vi "main_control_combo_reframe.vi"() -> ()   [LabVIEW 2019]
doc: "The Basic Serial Read and Write example performs a Serial Port Read, a Serial Port Write, or a combination of these actions. The user selects the actions (read or write) on the front panel. If both are selected, the VI will write the data first, read data, and then close the VISA session that is opened to the port. This VI will wait until the specified number of bytes is received at the port. Only the number of bytes specified will be read.\n\nINSTRUCTIONS:\n1) Select the serial resource and configuration parameters (baud rate, data bits, parity, stop bits, flow control).\n2) Select the operations to be performed. \n3) Connect the serial port to your device. If no device is available, perform a loopback test by doing one of the following. Short pins 2 and 3 on a RS-232 cable or short pin 4 to pin 8 and pin 5 to pin 9 on a RS-485/422 cable. \n4) Run the VI to see the data read. (The \"read string\" will match the \"string to write\" if a loopback test was performed.)\n\nNote: The parameters set for the serial port must match the parameters of the connected instrument or device. In this example, the bytes to read parameter specifies the number of bytes that the serial port reads. If there were more bytes at the port than the number specified in bytes to read, those bytes would not be read. Also, if you specify to read more bytes than the number of bytes actually read, you might receive a timeout error message.\n\nOn the block diagram, the Configure Serial Port VI sets the configuration parameters. The front panel displays the controls used to configure the basic parameters, such as baud rate, data bits, and parity. Constants configure the other parameters the user probably does not need set. After the VISA Configure Serial Port VI opens the VISA session and configures the port, the VI passes the VISA resource name to other VIs that perform operations on that VISA resource. The VISA Write function sends a command to the serial device and the VISA Read function returns data based on the command. The VISA Close function then closes the reference to the serial device. It is important to close the reference; otherwise communication through with that port through protocols other than VISA might not be possible."
uses:
  <vilib>/Instr/_visa.llb/VISA Configure Serial Port (Instr).vi
  <vilib>/Utility/file.llb/Read Delimited Spreadsheet (string).vi
  Keithley/Keithley 24XX/Public/Data/Read (Single Point).vi
  Keithley/Keithley 24XX/Keithley 24XX.lvlib
  <resource>/objmgr/ni.var.rc
panel:
  in  "Times to Run":i32
  out "DeltaPS output voltage":string
  out "SEH LV PS actual voltage":string
  out "Inverter PS actual voltage":string
  out "chiller actual temperature":string
  out "COMBO COMMAND":string
  in  "stop reading script":bool
  out "concatenated string":string
  out "dewpoint":string
  out "temperature":string
  out "humidity":string
  out "n2 flow temperature":string
  out "dewpoint":string
  out "From Linux Box":string
  in  "Voltage Manual Range (1.0) 2":dbl=1.0
  in  "Current Manual Range (1.0) 2":dbl=1.0
  in  "Resistance Manual Range (1.0) 2":dbl=1.0
  in  "Enable Voltage Auto Range (T:Enable) 2":bool=TRUE
  in  "Enable Current Auto Range (T:Enable) 2":bool=TRUE
  in  "Enable Resistance Auto Range (T:Enable) 2":bool=TRUE
  out "Voltage 3":sgl
  out "Current 3":sgl
  out "Resistance 2":sgl
  out "Current Micro 2":sgl
  out "Command Log and Output":string
  out "all rows":string[][](array[string])
  out "current command":string[](array[string])
  in  "file path (dialog if empty) 2":path
  in  "Read Script":bool
  out "relay TTi":errorcluster
  out "LV TTi":errorcluster
  out "Chiller":errorcluster
  out "N2 temperature > dew point + 2C":bool
  in  "File Path of rotonic datalog":path
  out "time humidity temporature dewpoint":string[](array[string])
  in  "Quit":bool
  # "Keithley Powersupply"
  # "µA"
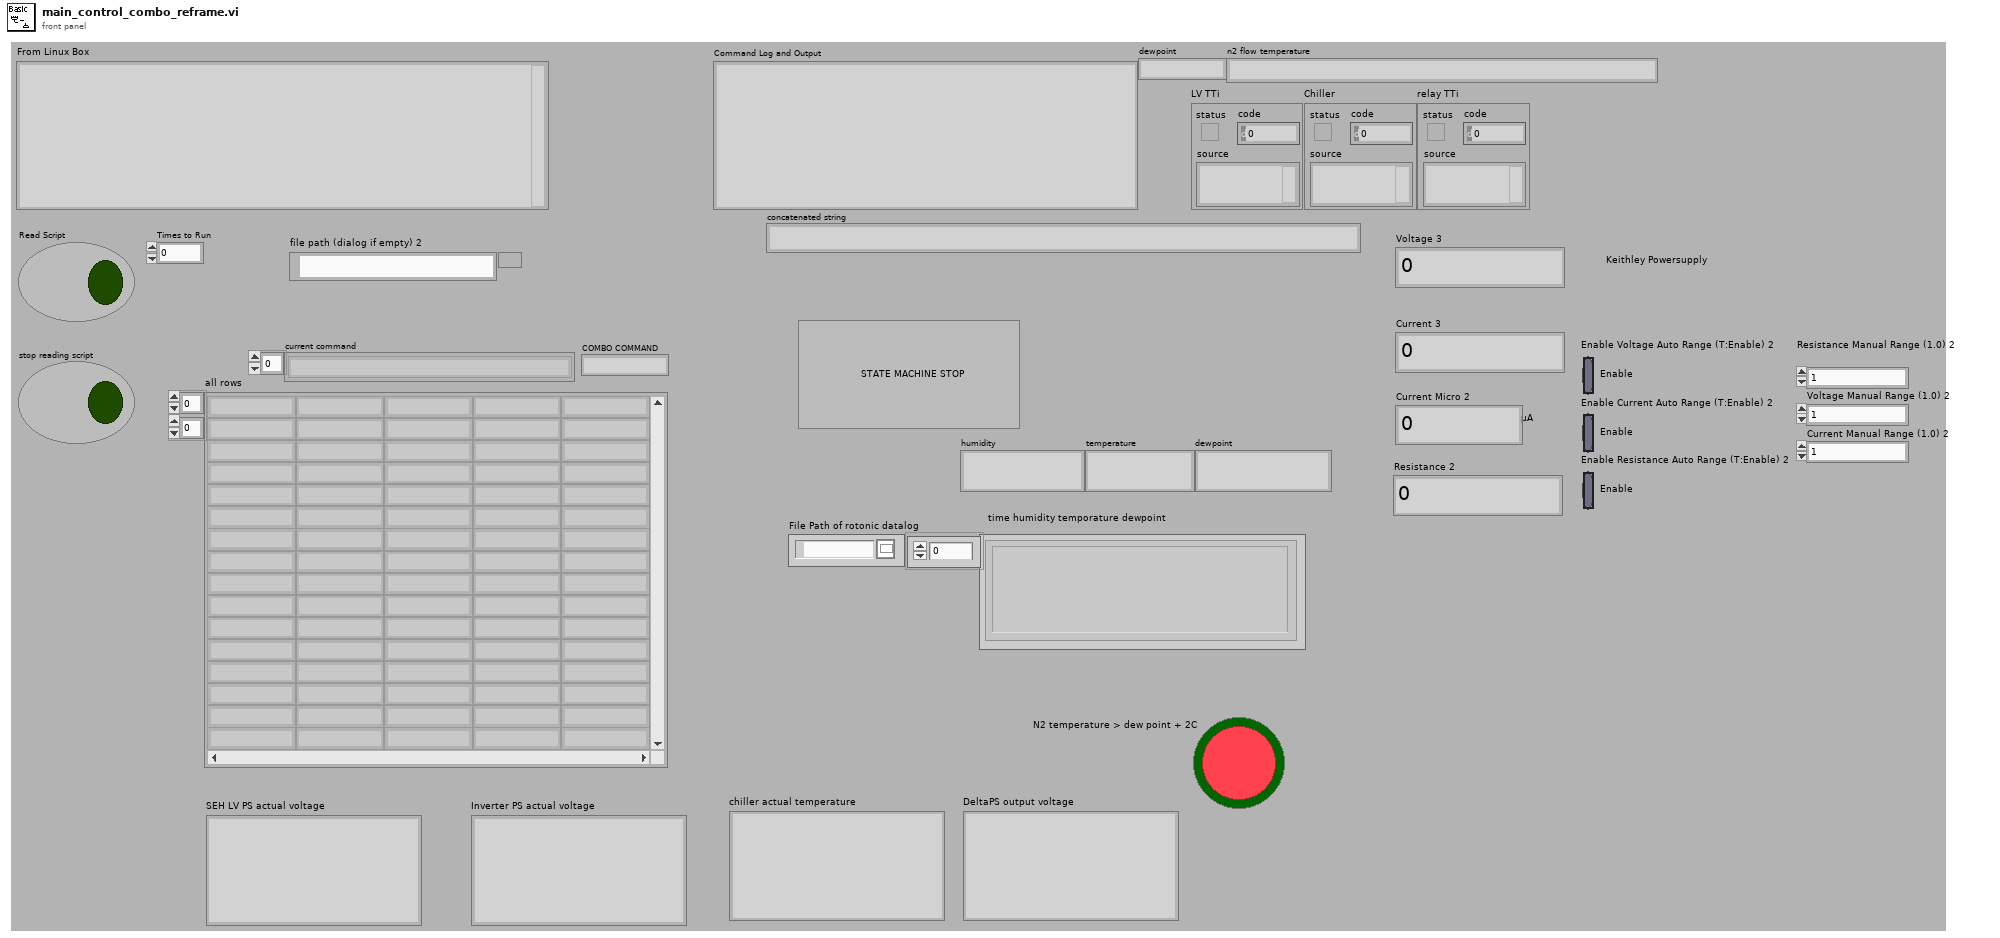
[diagram p1: front panel]
types:
  T1 = cluster{"Baud Rate":u32, "Parity":u16, "Data Bits":u16, "Stop Bits":u16, "Flow Control":u16}
  T2 = enum16{"open", "replace", "create", "open or create", "replace or create", "replace or create with confirmation"}
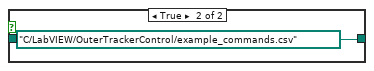
[diagram p2: hidden frame]
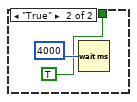
[diagram p3: hidden frame]
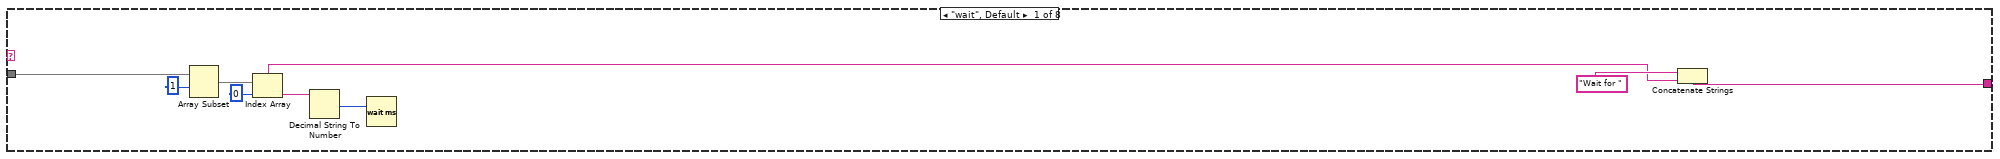
[diagram p5: hidden frame]
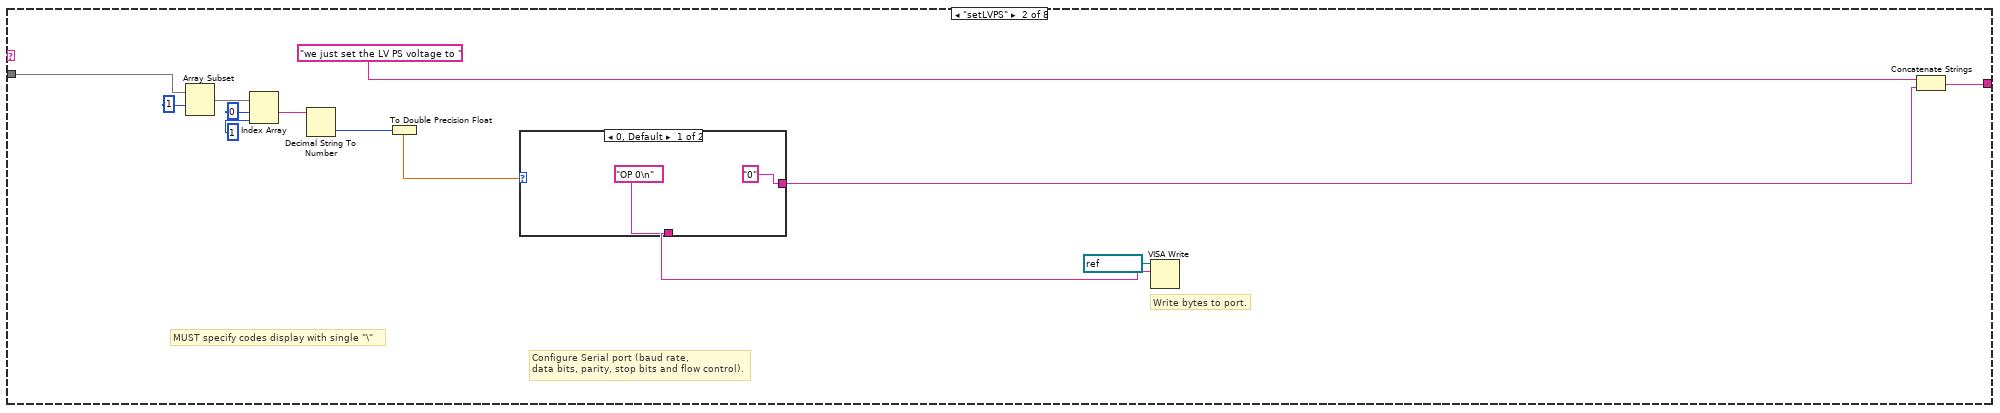
[diagram p6: hidden frame]
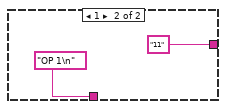
[diagram p7: hidden frame]
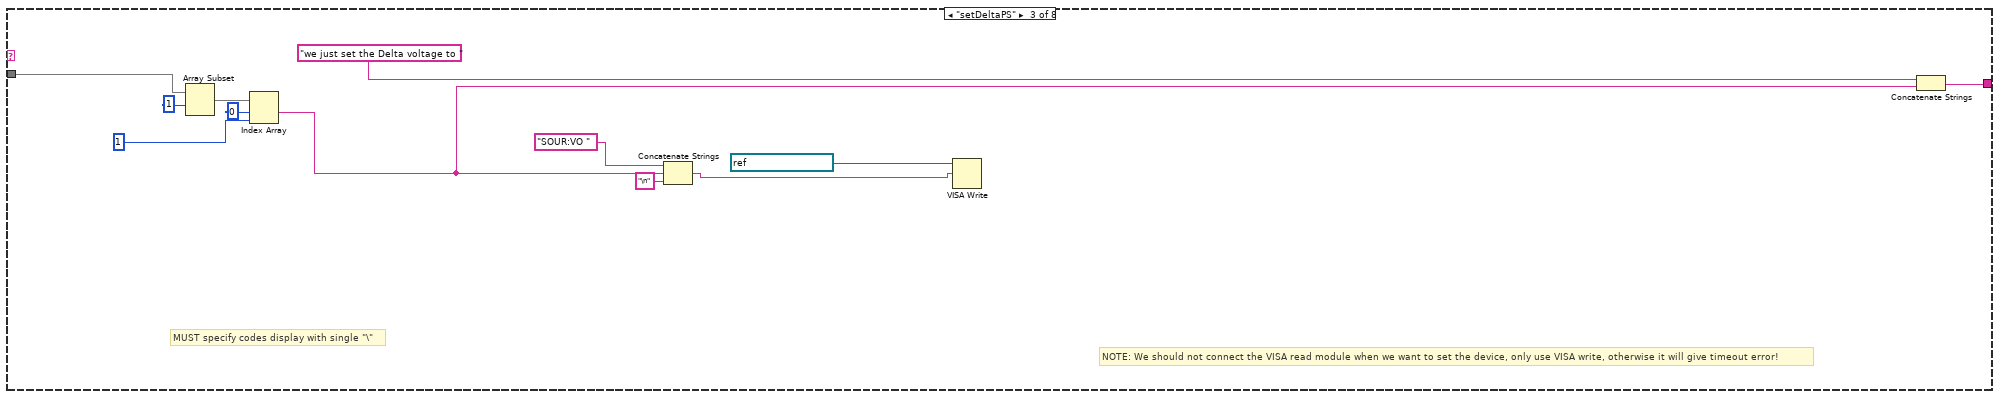
[diagram p8: hidden frame]
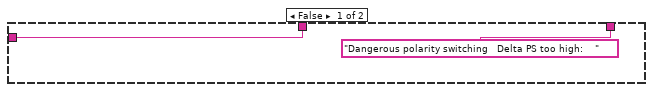
[diagram p9: hidden frame]
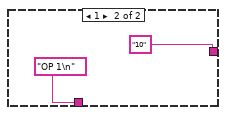
[diagram p10: hidden frame]
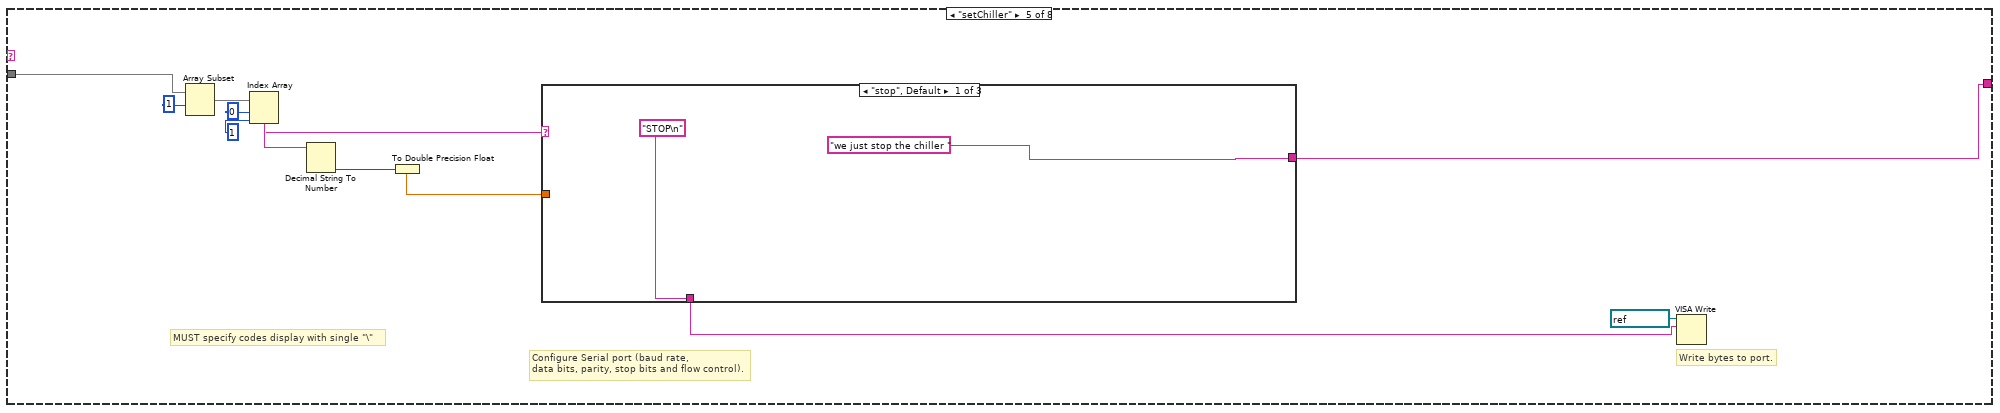
[diagram p11: hidden frame]
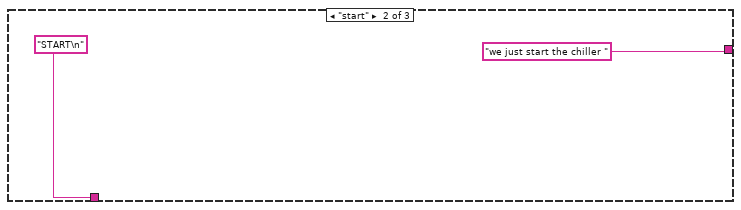
[diagram p12: hidden frame]
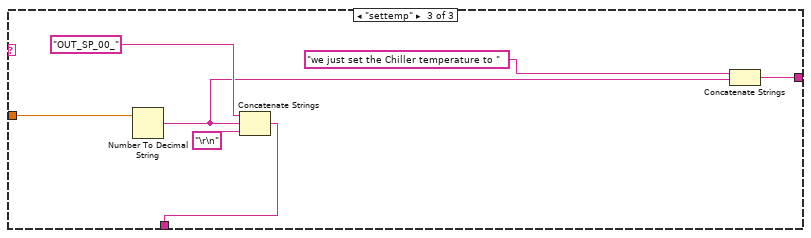
[diagram p13: hidden frame]
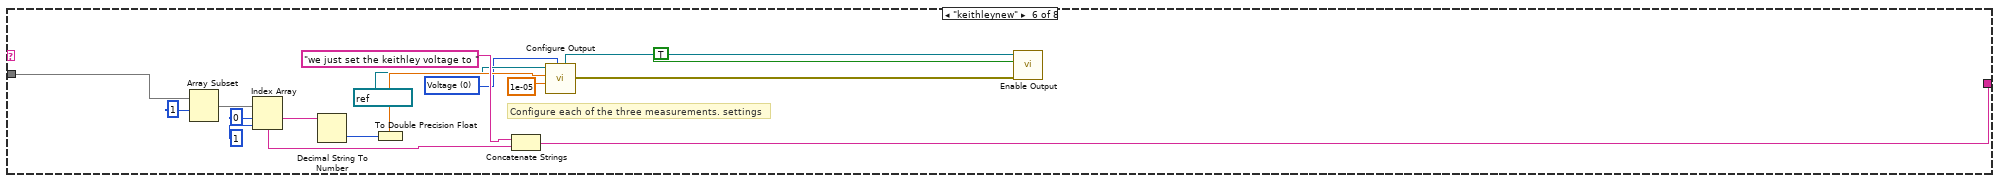
[diagram p14: hidden frame]
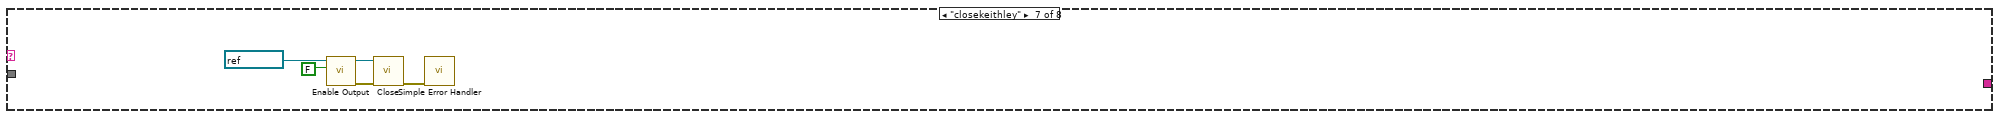
[diagram p15: hidden frame]
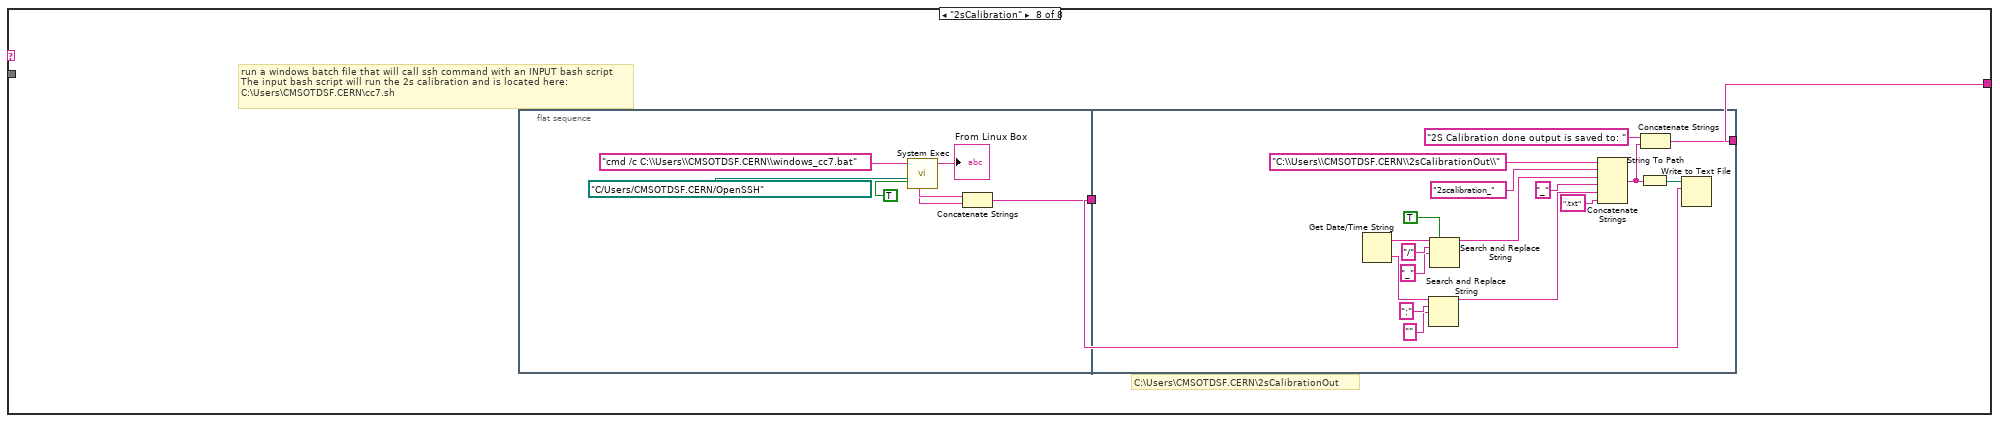
[diagram p16: hidden frame]
diagram:
  # "First save permanent values in non-volatile memory via NI - Max and the *SAV after setting it via SO:VO:MA 52 and SO:CU:MA 30    !"
  n1 = flat-sequence {
    tunnel: [w37] -> w16
    tunnel: [w36] -> w15
    tunnel: [w28] -> w14
    tunnel: [w27] -> w13
    tunnel: [w23] -> w12
    tunnel: [w22] -> w11
    tunnel: [w19] -> w10
    tunnel: [w18] -> w9
    tunnel: w16 -> [w44]
    tunnel: w15 -> [w45]
    tunnel: w14 -> [w43]
    tunnel: w13 -> [w42]
    tunnel: w12 -> [w46]
    tunnel: w11 -> [w47]
    tunnel: w10 -> [w41]
    tunnel: w9 -> [w40]
    tunnel: [w47] -> w8
    tunnel: [w46] -> w7
    tunnel: [w45] -> w6
    tunnel: [w44] -> w5
    tunnel: [w43] -> w4
    tunnel: [w42] -> w3
    tunnel: [w41] -> w2
    tunnel: [w40] -> w1
    tunnel: w8 -> [w359]
    tunnel: w7 -> [w358]
    tunnel: w6 -> [w357]
    tunnel: w5 -> [w356]
    tunnel: w4 -> [w355]
    tunnel: w3 -> [w354]
    tunnel: w2 -> [w353]
    tunnel: w1 -> [w352]
    frame #0 {
      w20 = u32 500  # timeout (10sec)
      w24 = FALSE  # Enable Termination Char (T)
      w25 = u32 3000  # timeout (10sec)
      w29 = FALSE  # Enable Termination Char (T)
      w30 = u32 3000  # timeout (10sec)
      w35 = u32 3000  # timeout (10sec)
      w33 = FALSE  # Enable Termination Char (T)
      n2 = call "Initialize.vi"("Serial Configuration"=T1 {"Baud Rate"=9600, "Parity"=0, "Data Bits"=8, "Stop Bits"=10, "Flow Control"=1}, "Reset (True)"=FALSE, "VISA resource name"=refnum<visa-resource-name> "COM1" ("VISA resource name 4")) -> ()  [unwired: 7 in, 2 out]
      n3 = call-poly "VISA Configure Serial Port"("VISA resource name"=refnum<visa-resource-name> "COM4", "timeout (10sec)"=w35, "Enable Termination\nChar (T)"=w33) -> ("VISA resource name out"=w36:refnum<visa-resource-name>, "error out"=w37:errorcluster)  [unwired: 11 in]
      n4 = VISA Open(timeout (0)=w20, VISA resource name=refnum<visa-resource-name> "GPIB0::8::INSTR") -> (VISA resource name=w19:refnum<visa-resource-name>, error out=w18:errorcluster)  [unwired: 3 in]
      n5 = call-poly "VISA Configure Serial Port"("VISA resource name"=refnum<visa-resource-name> "COM5", "timeout (10sec)"=w25, "Enable Termination\nChar (T)"=w24) -> ("VISA resource name out"=w22:refnum<visa-resource-name>, "error out"=w23:errorcluster)  [unwired: 11 in]
      n6 = call-poly "VISA Configure Serial Port"("VISA resource name"=refnum<visa-resource-name> "COM6", "timeout (10sec)"=w30, "Enable Termination\nChar (T)"=w29) -> ("VISA resource name out"=w28:refnum<visa-resource-name>, "error out"=w27:errorcluster)  [unwired: 11 in]
    }
    frame #1 {
      # "Disable Output"
      # "State machine for iterating through commands from table"
      n7 = while {
        stop <- w94 stop-if-true
        n8 = local read "Quit"() -> (w94:bool)
        n9 = case shown="True" "Read Script" {
          tunnel: "Times to Run" -> [_ w99]
          frame False {
          }
          frame True {
            n10 = Get Date/Time String() -> (date string=w122:string, time string=w120:string)  [unwired: 3 in]
            n11 = Search and Replace String(replace all?=TRUE ("replace all? (F)"), input string=w122, search string="/", replace string="_" ("replace string (\"\")")) -> (result string=w121:string)  [unwired: 4 in, 3 out]
            n12 = Search and Replace String(input string=w120, search string=":", replace string="" ("replace string (\"\")")) -> (result string=w119:string)  [unwired: 5 in, 3 out]
            n13 = Concatenate Strings("C:\\Users\\CMSOTDSF.CERN\\ExecutedCommands\\" ("string"), "command_log_" ("string"), w121, "_" ("string"), w119, ".txt" ("string")) -> (w118:string)
            n14 = String To Path(string=w118) -> (path=w108:path)
            n15 = Open/Create/Replace File(file path (use dialog)=w108, operation (0:open)=T2."replace or create") -> (refnum out=w107:refnum<file>)  [unwired: 4 in, 2 out]
            n16 = Concatenate Strings("Command Log Header for Executed CSV commands " ("text"), "\r\n") -> (w100:string)
            n17 = Set File Position(offset (in bytes) (0)=i64 0, refnum=w107, from (0:start)=enum16{"start", "end", "current"}."end") -> (refnum out=w104:refnum<file>)  [unwired: 1 in, 1 out]
            n18 = Write to Text File(file (use dialog)=w104, text=w100) -> ()  [unwired: 2 in, 3 out]
            n19 = call-poly <vilib>:"Read Delimited Spreadsheet.vi"("file path (dialog if empty)"="file path (dialog if empty) 2", "delimiter (\\t)"="," ("delimiter (\\t)")) -> ("all rows"=w97:string[][])  [unwired: 8 in, 5 out]
            n20 = flat-sequence {
              tunnel: w108 -> [w125]
              tunnel: w99 -> [w124]
              tunnel: w97 -> [w123]
              frame #0 {
                n21 = for {
                  N: w124 -> [_]
                  tunnel: w125 -> [w131]
                  tunnel: w123 -> [w130]
                  # "read table from CSV"
                  n22 = Array Size(array=w130) -> (size(s)=w128:i32[])
                  n23 = Index Array(array=w128, index #1=0 ("index"), index #2=1 ("index")) -> (element #1=w129:i32)  [unwired: 1 out]
                  n24 = for {
                    N: w129 -> [_]
                    tunnel: w130 -> [w137] mode=indexing
                    tunnel: w131 -> [w133]
                    i -> [w132]
                    stop <- w134 stop-if-true
                    n25 = flat-sequence {
                      tunnel: w137 -> [w158]
                      tunnel: w133 -> [w149]
                      tunnel: w132 -> [w146]
                      frame #0 {
                        n26 = Array Subset(array=w158) -> (w155:string[])  [unwired: 2 in]
                        "current command" <- w155
                        n27 = Array Size(array=w155) -> (size(s)=w157:i32)
                        n28 = Index Array(array=w155, index=0) -> (element=w138:string)
                        n29 = local write "COMBO COMMAND"(w138) -> ()
                        n30 = for {
                          N: w157 -> [_]
                          tunnel: w155 -> [w295]
                          tunnel: [w296] -> w139 mode=indexing
                          i -> [w298]
                          n31 = Add(x=w298, y=1) -> (x+y=w294:i32)
                          n32 = Wait Until Next ms Multiple(millisecond multiple=u32 1000) -> ()  [unwired: 1 out]
                          n33 = Index Array(array=w295, index=w294) -> (element=w293:string)
                          n34 = Concatenate Strings(w293, "   " ("string")) -> (w296:string)
                        }
                        n35 = case shown="\"setInverter\"" w138 {
                          tunnel: w155 -> [w166 w174 w191 w206 w230 w258 _ _]
                          tunnel: [w160 w171 w189 w204 w223 w254 _ w267] -> w147
                          frame "wait", Default {
                            n36 = Array Subset(array=w166, index=1) -> (w164:string[])  [unwired: 1 in]
                            n37 = Index Array(array=w164, index=0) -> (element=w161:string)
                            n38 = Decimal String To Number(string=w161) -> (number=w159:i32)  [unwired: 2 in, 1 out]
                            n39 = Wait (ms)(milliseconds to wait=w159) -> ()  [unwired: 1 out]
                            n40 = Concatenate Strings("Wait for ", w161) -> (w160:string)
                          }
                          frame "setLVPS" {
                            # "Write bytes to port."
                            # "MUST specify codes display with single \"\\\""
                            # "Configure Serial port (baud rate,\ndata bits, parity, stop bits and flow control)."
                            n41 = Array Subset(array=w174, index=1) -> (w179:string[])  [unwired: 1 in]
                            n42 = Index Array(array=w179, index #1=0 ("index"), index #2=1 ("index")) -> (element #1=w176:string)  [unwired: 1 out]
                            n43 = Decimal String To Number(string=w176) -> (number=w173:i32)  [unwired: 2 in, 1 out]
                            n44 = To Double Precision Float(number=w173) -> (double precision float=w170:dbl)
                            n45 = case shown="0, Default" w170 {
                              tunnel: ["OP 0\n" ("Combo Box 4") "OP 1\n" ("Combo Box 4")] -> w169
                              tunnel: ["0" ("Combo Box 4") "11" ("Combo Box 4")] -> w167
                              frame 0, Default {
                              }
                              frame 1 {
                              }
                            }
                            n46 = VISA Write(VISA resource name=refnum<visa-resource-name> "COM5", write buffer=w169) -> ()  [unwired: 1 in, 3 out]
                            n47 = Concatenate Strings("we just set the LV PS voltage to ", w167) -> (w171:string)
                          }
                          frame "setDeltaPS" {
                            # "NOTE: We should not connect the VISA read module when we want to set the device, only use VISA write, otherwise it will give timeout error!"
                            # "MUST specify codes display with single \"\\\""
                            n48 = Array Subset(array=w191, index=1) -> (w195:string[])  [unwired: 1 in]
                            n49 = Index Array(array=w195, index #1=0 ("index"), index #2=1 ("index")) -> (element #1=w184:string)  [unwired: 1 out]
                            n50 = Concatenate Strings("SOUR:VO " ("format string"), w184, "\n" ("string")) -> (w186:string)
                            n51 = VISA Write(VISA resource name=refnum<visa-resource-name> "GPIB0::8::INSTR", write buffer=w186) -> ()  [unwired: 1 in, 3 out]
                            n52 = Concatenate Strings("we just set the Delta voltage to ", w184) -> (w189:string)
                          }
                          frame "setInverter" {
                            # "MUST specify codes display with single \"\\\""
                            # "Configure Serial port (baud rate,\ndata bits, parity, stop bits and flow control)."
                            n53 = Array Subset(array=w206, index=1) -> (w211:string[])  [unwired: 1 in]
                            n54 = Index Array(array=w211, index #1=0 ("index"), index #2=1 ("index")) -> (element #1=w208:string)  [unwired: 1 out]
                            n55 = Decimal String To Number(string=w208) -> (number=w205:i32)  [unwired: 2 in, 1 out]
                            n56 = To Double Precision Float(number=w205) -> (double precision float=w201:dbl)
                            n57 = call "deltaPS.vi"("VISA Refnum in"=refnum<visa-resource-name> "GPIB0::8::INSTR" ("VISA resource name")) -> ("DeltaPS"=w196:string)  [unwired: 10 in]
                            n58 = Decimal String To Number(string=w196) -> (number=w197:i32)  [unwired: 2 in, 1 out]
                            n59 = Less?(x=w197, y=3.0) -> (x < y?=w202:bool)
                            n60 = case shown="True" w202 {
                              tunnel: w201 -> [_ w216]
                              tunnel: [w212 w215] -> w200
                              tunnel: ["Dangerous polarity switching   Delta PS too high:    " "we just set the Inverter voltage to "] -> w199
                              tunnel: w196 -> [w212 _]
                              frame False {
                              }
                              frame True {
                                # "Write bytes to port."
                                n61 = case shown="0, Default" w216 {
                                tunnel: ["OP 0\n" ("Combo Box 4") "OP 1\n" ("Combo Box 4")] -> w218
                                tunnel: ["0" ("Combo Box 4") "10" ("Combo Box 4")] -> w215
                                frame 0, Default {
                                }
                                frame 1 {
                                }
                                }
                                n62 = VISA Write(VISA resource name=refnum<visa-resource-name> "COM4", write buffer=w218) -> ()  [unwired: 1 in, 3 out]
                              }
                            }
                            n63 = Concatenate Strings(w199, w200) -> (w204:string)
                          }
                          frame "setChiller" {
                            # "Write bytes to port."
                            # "MUST specify codes display with single \"\\\""
                            # "Configure Serial port (baud rate,\ndata bits, parity, stop bits and flow control)."
                            n64 = Array Subset(array=w230, index=1) -> (w234:string[])  [unwired: 1 in]
                            n65 = Index Array(array=w234, index #1=0 ("index"), index #2=1 ("index")) -> (element #1=w225:string, element #2=w227:string)
                            n66 = Decimal String To Number(string=w227) -> (number=w226:i32)  [unwired: 2 in, 1 out]
                            n67 = To Double Precision Float(number=w226) -> (double precision float=w224:dbl)
                            n68 = case shown="\"stop\", Default" w225 {
                              tunnel: ["STOP\n" ("Combo Box 4") "START\n" ("Combo Box 4") w243] -> w229
                              tunnel: w224 -> [_ _ w242]
                              tunnel: ["we just stop the chiller " "we just start the chiller " w240] -> w223
                              frame "stop", Default {
                              }
                              frame "start" {
                              }
                              frame "settemp" {
                                n69 = Number To Decimal String(number=w242) -> (decimal integer string=w239:string)  [unwired: 1 in]
                                n70 = Concatenate Strings("OUT_SP_00_" ("Combo Box 4"), w239, "\r\n" ("string")) -> (w243:string)
                                n71 = Concatenate Strings("we just set the Chiller temperature to ", w239) -> (w240:string)
                              }
                            }
                            n72 = VISA Write(VISA resource name=refnum<visa-resource-name> "COM6", write buffer=w229) -> ()  [unwired: 1 in, 3 out]
                          }
                          frame "keithleynew" {
                            w246 = u16 0 items=["Voltage", "Current"] ("Source Mode  (0: Voltage)")
                            # "Configure each of the three measurements. settings"
                            n73 = Array Subset(array=w258, index=1) -> (w261:string[])  [unwired: 1 in]
                            n74 = Index Array(array=w261, index #1=0 ("index"), index #2=1 ("index")) -> (element #1=w255:string)  [unwired: 1 out]
                            n75 = Decimal String To Number(string=w255) -> (number=w257:i32)  [unwired: 2 in, 1 out]
                            n76 = To Double Precision Float(number=w257) -> (double precision float=w252:dbl)
                            n77 = Concatenate Strings("we just set the keithley voltage to ", w255) -> (w254:string)
                            n78 = call "Configure Output.vi"("Source Mode  (0: Voltage)"=w246, "Compliance  Level (0.1)"=1e-05, "Output Level (0)"=w252, "VISA resource name"=refnum<visa-resource-name> "COM1") -> ("error out"=w250:errorcluster, "VISA resource name out"=w251:refnum<visa-resource-name>)  [unwired: 6 in]
                            n79 = call "Enable Output.vi"("error in (no error)"=w250, "Enable Output (T: Enable)"=TRUE, "VISA resource name"=w251) -> ()  [unwired: 7 in, 2 out]
                          }
                          frame "closekeithley" {
                            n80 = call "Enable Output.vi"("Enable Output (T: Enable)"=FALSE, "VISA resource name"=refnum<visa-resource-name> "COM1") -> ("error out"=w263:errorcluster, "VISA resource name out"=w264:refnum<visa-resource-name>)  [unwired: 8 in]
                            n81 = call "Close.vi"("error in (no error)"=w263, "VISA resource name"=w264) -> ("error out"=w266:errorcluster)  [unwired: 9 in]
                            n82 = call <vilib>:"Simple Error Handler.vi"("error in (no error)"=w266) -> ()  [unwired: 4 in, 5 out]
                          }
                          frame "2sCalibration" {
                            # "C:\\Users\\CMSOTDSF.CERN\\2sCalibrationOut"
                            # "run a windows batch file that will call ssh command with an INPUT bash script\nThe input bash script will run the 2s calibration and is located here:\nC:\\Users\\CMSOTDSF.CERN\\cc7.sh"
                            n83 = flat-sequence {
                              tunnel: [w270] -> w268
                              tunnel: w268 -> [w276]
                              tunnel: [w275] -> w267
                              frame #0 {
                                n84 = call <vilib>:"System Exec.vi"("run minimized? (F)"=TRUE, "working directory"=path "C:/Users/CMSOTDSF.CERN/OpenSSH", "command line"="cmd /c C:\\Users\\CMSOTDSF.CERN\\windows_cc7.bat") -> ("standard error"=w271:string, "standard output"=w272:string)  [unwired: 5 in, 2 out]
                                "From Linux Box" <- w272
                                n85 = Concatenate Strings(w272, w271) -> (w270:string)
                              }
                              frame #1 {
                                n86 = Get Date/Time String() -> (date string=w287:string, time string=w289:string)  [unwired: 3 in]
                                n87 = Search and Replace String(input string=w289, search string=":", replace string="" ("replace string (\"\")")) -> (result string=w290:string)  [unwired: 5 in, 3 out]
                                n88 = Search and Replace String(replace all?=TRUE ("replace all? (F)"), input string=w287, search string="/", replace string="_" ("replace string (\"\")")) -> (result string=w288:string)  [unwired: 4 in, 3 out]
                                n89 = Concatenate Strings("C:\\Users\\CMSOTDSF.CERN\\2sCalibrationOut\\" ("string"), "2scalibration_" ("string"), w288, "_" ("string"), w290, ".txt" ("string")) -> (w291:string)
                                n90 = String To Path(string=w291) -> (path=w292:path)
                                n91 = Concatenate Strings("2S Calibration done output is saved to: ", w291) -> (w275:string)
                                n92 = Write to Text File(file (use dialog)=w292, text=w276) -> ()  [unwired: 2 in, 3 out]
                              }
                            }
                          }
                        }
                        "Command Log and Output" <- w147
                        n93 = Add(x=w146, y=1) -> (x+y=w144:i32)
                        n94 = Number To Decimal String(number=w144) -> (decimal integer string=w143:string)  [unwired: 1 in]
                        n95 = Open/Create/Replace File(file path (use dialog)=w149, operation (0:open)=T2."open") -> (refnum out=w150:refnum<file>)  [unwired: 4 in, 2 out]
                        n96 = Concatenate Strings(w143, "  " ("string"), w138, "  " ("string"), w139, "\r\n") -> (w148:string)
                        n97 = Set File Position(offset (in bytes) (0)=i64 0, refnum=w150, from (0:start)=enum16{"start", "end", "current"}."end") -> (refnum out=w152:refnum<file>)  [unwired: 1 in, 1 out]
                        n98 = Write to Text File(file (use dialog)=w152, text=w148) -> ()  [unwired: 2 in, 3 out]
                      }
                      frame #1 {
                        n99 = call "TTiPS.vi"("VISA Refnum in"=refnum<visa-resource-name> "COM5") -> ("TTi PS actual voltage"=→"SEH LV PS actual voltage":string)  [unwired: 10 in]
                        n100 = call "TTiPS.vi"("VISA Refnum in"=refnum<visa-resource-name> "COM4") -> ("TTi PS actual voltage"=→"Inverter PS actual voltage":string)  [unwired: 10 in]
                        n101 = call "chiller.vi"("VISA Refnum in"=refnum<visa-resource-name> "COM6" ("VISA resource name")) -> ("chiller actual temperature"=→"chiller actual temperature":string)  [unwired: 10 in]
                        n102 = call "deltaPS.vi"("VISA Refnum in"=refnum<visa-resource-name> "GPIB0::8::INSTR" ("VISA resource name")) -> ("DeltaPS"=→"DeltaPS output voltage":string)  [unwired: 10 in]
                      }
                    }
                    n103 = local read "Quit"() -> (w136:bool)
                    n104 = Or(x=w136, y="stop reading script") -> (x .or. y?=w134:bool)
                  }
                  "all rows" <- w130
                }
              }
              frame #1 {
                n105 = invoke on="Read Script" class="Bool (strict)" method="Reinit To Default"() -> ()  [unwired: 3 in, 3 out]
                n106 = local write "COMBO COMMAND"("" ("COMBO COMMAND")) -> ()
              }
            }
          }
        }
      }
      n107 = while {
        tunnel: ["Quit"] -> _
        stop <- "Quit" stop-if-true
      }
      n108 = while {
        stop <- w49 stop-if-true
        n109 = local read "file path (dialog if empty) 2"() -> (w50:path)
        n110 = Equal?(x=w50, y=path "") -> (x = y?=w54:bool)
        n111 = case shown="False" w54 {
          tunnel: [w56 path "C:/LabVIEW/OuterTrackerControl/example_commands.csv"] -> w55
          tunnel: w50 -> [w56 _]
          frame False {
          }
          frame True {
          }
        }
        n112 = local read "Quit"() -> (w49:bool)
        n113 = call-poly <vilib>:"Read Delimited Spreadsheet.vi"("file path (dialog if empty)"=w55, "delimiter (\\t)"="," ("delimiter (\\t)")) -> ("all rows"=w53:string[][])  [unwired: 8 in, 5 out]
        n114 = local write "all rows"(w53) -> ()
      }
      n115 = while {
        stop <- w310 stop-if-true
        (unwired) "humidity_202105"
        (unwired) path "C:/Users/fengwang.PCCMSTKUPDSF2/Desktop/RotronicUSBDriver/dataLog" ("file (use dialog)")
        # "dew point"
        # "N2 flow temperature"
        # "Convert text file string to array"
        # "Return the Number of lines."
        # "Extract only the size dimension we need"
        # "Get the size of the array"
        # "Read Text File, dialog box if none"
        n116 = local read "Quit"() -> (w310:bool)
        n117 = Get Date/Time In Seconds() -> (seconds since 1Jan1904=w316:timestamp)
        n118 = Format Date/Time String(time format string (%c)="%d_%m_%Y", seconds (now)=w316) -> (date/time string=w314:string)  [unwired: 1 in]
        n119 = Concatenate Strings("C:\\Users\\fengwang.PCCMSTKUPDSF2\\Desktop\\RotronicUSBDriver\\dataLog\\humidity_", w314) -> (→"concatenated string":string)
        n120 = Read from Text File(file (use dialog)="File Path of rotonic datalog") -> (text=w343:string)  [unwired: 1 in, 5 out]
        n121 = Spreadsheet String To Array(delimiter (Tab)="\r", format string="%d", spreadsheet string=w343) -> (array=w341:dbl[][])  [unwired: 1 out]
        n122 = Array Size(array=w341) -> (size(s)=w342:i32[])
        n123 = Index Array(array=w342) -> (element=w345:i32)  [unwired: 1 in]
        n124 = Read from Text File(file (use dialog)="File Path of rotonic datalog", count=w345) -> (text=w346:string[])  [unwired: 1 in, 4 out]
        n125 = Decrement(x=w345) -> (x-1=w344:i32)
        n126 = Array Subset(array=w346, index=w344) -> (w347:string[])  [unwired: 1 in]
        "time humidity temporature dewpoint" <- w347
        n127 = Get Date/Time In Seconds() -> (seconds since 1Jan1904=w339:timestamp)
        n128 = Array To Spreadsheet String(array=w347, 3:"%d/%m/%Y %H:%M:%S %4.12f %4.12f %4.12f" ("time format string (%c)")) -> (spreadsheet string=w318:string)  [unwired: 1 in]
        n129 = Format Date/Time String(time format string (%c)="%d/%m/%Y %H:%M:%S ", seconds (now)=w339) -> (date/time string=w340:string)  [unwired: 1 in]
        n130 = String Subset(string=w318, offset (0)=20, length (rest)=5 ("length (rest)")) -> (substring=→"humidity":string)
        n131 = Scan From String(format string=w340, input string=w318) -> (remaining string=w348:string)  [unwired: 4 in, 2 out]
        n132 = String Subset(string=w318, offset (0)=27, length (rest)=5 ("length (rest)")) -> (substring=→"temperature":string)
        n133 = String Subset(string=w318, offset (0)=34, length (rest)=6 ("length (rest)")) -> (substring=w311:string)
        "dewpoint" <- w311
        n134 = property class="Variable Object" props=["ClassId"](reference=w311) -> ()  [unwired: 1 in, 3 out]
        n135 = String Subset(string=w348, offset (0)=12, length (rest)=5 ("length (rest)")) -> (substring=w349:string)
        "dewpoint" <- w349
        n136 = Fract/Exp String To Number(string=w349) -> (number=w329:dbl)  [unwired: 3 in, 1 out]
        n137 = String Subset(string=w348, offset (0)=6, length (rest)=5 ("length (rest)")) -> (substring=w327:string)
        "n2 flow temperature" <- w327
        n138 = Fract/Exp String To Number(string=w327) -> (number=w350:dbl)  [unwired: 3 in, 1 out]
        n139 = Add(x=w329, y=2.0) -> (x+y=w328:dbl)
        n140 = Greater?(x=w350, y=w328) -> (0:→"N2 temperature > dew point + 2C":bool)
        n141 = call <vilib>:"Simple Error Handler.vi"() -> ()  [unwired: 5 in, 5 out]
      }
      n142 = while {
        stop <- w61 stop-if-true
        w76 = u16 0 items=["Volts", "Current", "Resistance"]  # Function (0: Volts)
        w83 = u16 2 items=["Volts", "Current", "Resistance"]  # Function (0: Volts)
        w84 = u16 1 items=["Volts", "Current", "Resistance"]  # Function (0: Volts)
        # "Take the readings."
        # "Configure the output."
        # "Configure each of the three measurements. settings"
        n143 = call "Configure Measurement.vi"("Manual Range (1.0)"="Voltage Manual Range (1.0) 2", "Enable Auto Range (T:Enable)"="Enable Voltage Auto Range (T:Enable) 2", "Function (0: Volts)"=w76, "VISA resource name"=refnum<visa-resource-name> "COM1") -> ("error out"=w87:errorcluster, "VISA resource name out"=w88:refnum<visa-resource-name>)  [unwired: 6 in]
        n144 = call "Configure Measurement.vi"("Manual Range (1.0)"="Current Manual Range (1.0) 2", "error in (no error)"=w87, "Enable Auto Range (T:Enable)"="Enable Current Auto Range (T:Enable) 2", "Function (0: Volts)"=w84, "VISA resource name"=w88) -> ("error out"=w86:errorcluster, "VISA resource name out"=w85:refnum<visa-resource-name>)  [unwired: 5 in]
        n145 = call "Configure Measurement.vi"("Manual Range (1.0)"="Resistance Manual Range (1.0) 2", "error in (no error)"=w86, "Enable Auto Range (T:Enable)"="Enable Resistance Auto Range (T:Enable) 2", "Function (0: Volts)"=w83, "VISA resource name"=w85) -> ("error out"=w65:errorcluster, "VISA resource name out"=w66:refnum<visa-resource-name>)  [unwired: 5 in]
        n146 = call "Enable Output.vi"("error in (no error)"=w65, "Enable Output (T: Enable)"=TRUE, "VISA resource name"=w66) -> ("error out"=w69:errorcluster, "VISA resource name out"=w68:refnum<visa-resource-name>)  [unwired: 7 in]
        n147 = local read "COMBO COMMAND"() -> (w58:string)
        n148 = call-poly "Read.vi"("VISA resource name"=w68, "error in (no error)"=w69) -> ("Voltage"=→"Voltage 3":sgl, "Current"=w74:sgl, "Resistance"=→"Resistance 2":sgl)  [unwired: 7 in, 4 out]
        "Current 3" <- w74
        n149 = Search and Replace String(input string=w58, search string="keithleynew", replace string="1" ("replace string (\"\")")) -> (result string=w62:string)  [unwired: 5 in, 3 out]
        n150 = Multiply(x=w74, y=sgl 1000000.0) -> (x*y=→"Current Micro 2":sgl)
        n151 = case shown="\"False\", Default" w62 {
          tunnel: [FALSE TRUE] -> w60
          frame "False", Default {
            n152 = Wait (ms)(milliseconds to wait=u32 4000) -> ()  [unwired: 1 out]
          }
          frame "True" {
            n153 = Wait (ms)(milliseconds to wait=u32 4000) -> ()  [unwired: 1 out]
          }
        }
        n154 = local read "Quit"() -> (w59:bool)
        n155 = Or(x=w59, y=w60) -> (x .or. y?=w61:bool)
      }
    }
    frame #2 {
      # "Closing things down"
      n156 = VISA Close(VISA resource name=w359, error in (no error)=w358) -> (error out=w360:errorcluster)
      "LV TTi" <- w360
      n157 = VISA Close(VISA resource name=w357, error in (no error)=w356) -> (error out=w361:errorcluster)
      "relay TTi" <- w361
      n158 = VISA Close(VISA resource name=w355, error in (no error)=w354) -> (error out=w362:errorcluster)
      "Chiller" <- w362
      n159 = VISA Close(VISA resource name=w353, error in (no error)=w352) -> ()  [unwired: 1 out]
      n160 = call <vilib>:"Simple Error Handler.vi"("error in (no error)"=w360) -> ()  [unwired: 4 in, 5 out]
      n161 = call <vilib>:"Simple Error Handler.vi"("error in (no error)"=w362) -> ()  [unwired: 4 in, 5 out]
      n162 = call <vilib>:"Simple Error Handler.vi"("error in (no error)"=w361) -> ()  [unwired: 4 in, 5 out]
    }
  }
  n163 = property on="dewpoint" class="Str"("Text.FontSize"=u32 30 ("Text.Font:Size")) -> ()  [unwired: 2 in, 2 out]
